vi "Driver Controller Global.vi"() -> ()   [LabVIEW 2018]
panel:
  in  "Rumble Amount":dbl=1.0
  out "Rumble Controller?":bool
  in  "Driver Right Trigger":dbl
  in  "Driver Left Trigger":dbl
  in  "Driver Right Stick Y":dbl
  in  "Driver Right Stick X":dbl
  in  "Driver Left Stick Y":dbl
  in  "Driver Left Stick X":dbl
  out "Driver Right Start":bool
  out "Driver Left Start":bool
  out "Driver Right Bumper":bool
  out "Driver Left Bumper":bool
  out "Driver Button Y":bool
  out "Driver Button X":bool
  out "Driver Button B":bool
  out "Driver Button A":bool
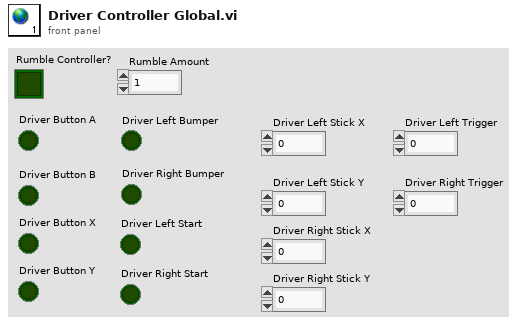
[diagram p1: front panel]
diagram:
